vi "json Member Names - array path.vi"(8 "error in (no error)":errorcluster, 10 "path":string[](array[string]), 11 "JSON Document in":refnum<class "JSON Document.lvclass">) -> (0 "error out":errorcluster, 2 "Member Names":string[](array[string]), 3 "JSON Document out":refnum<class "JSON Document.lvclass">)   [LabVIEW 2015, in "JSON Document.lvclass"]
uses:
  JSON Document.lvclass
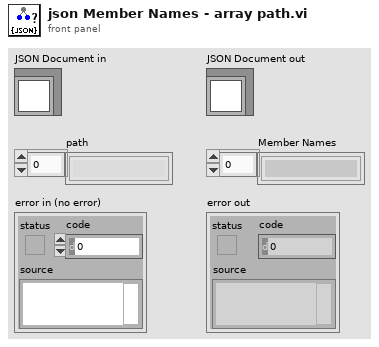
[diagram p1: front panel]
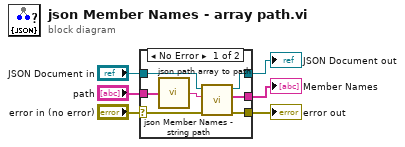
[diagram p0: block diagram]
diagram:
  n1 = case shown="No Error" "error in (no error)" {
    selector: "error in (no error)" -> [w7 w15]
    tunnel: [w8 w15] -> w5
    tunnel: [w10 w14] -> w3
    tunnel: "JSON Document in" -> [w11 w14]
    tunnel: "path" -> [w13 _]
    tunnel: [w9 _] -> w1
    frame No Error {
      n2 = call "json path array to path.vi"("path"=w13) -> ("String"=w12:string)
      n3 = call "json Member Names - string path.vi"("error in (no error)"=w7, "path"=w12, "JSON Document in"=w11) -> ("error out"=w8:errorcluster, "Member Names"=w9:string[], "JSON Document out"=w10:refnum<class "JSON Document.lvclass">)  [unwired: 6 in]
    }
    frame Error {
    }
  }
  "error out" <- w5
  "JSON Document out" <- w3
  "Member Names" <- w1
